vi "HowdyDrive.vi"(6 "highGear?":bool, 8 "error in (no error)":errorcluster, 9 "Y":dbl, 10 "X":dbl, 11 "Drive in":refnum<class "Drive.lvclass">) -> (0 "error out":errorcluster, 3 "Drive out":refnum<class "Drive.lvclass">)   [LabVIEW 2018, in "Drive.lvlib" / "Drive.lvclass"]
doc: "Runs motors based of joystick values in velocity closed loop mode, a version of arcade drive with support for CTRE motor controllers"
uses:
  Drive.lvclass
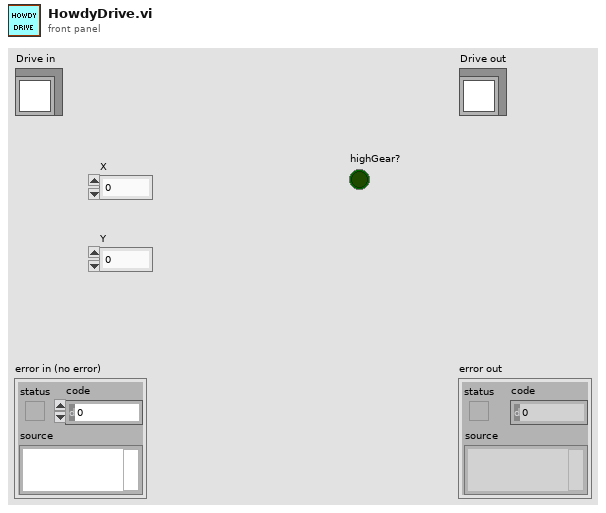
[diagram p1: front panel]
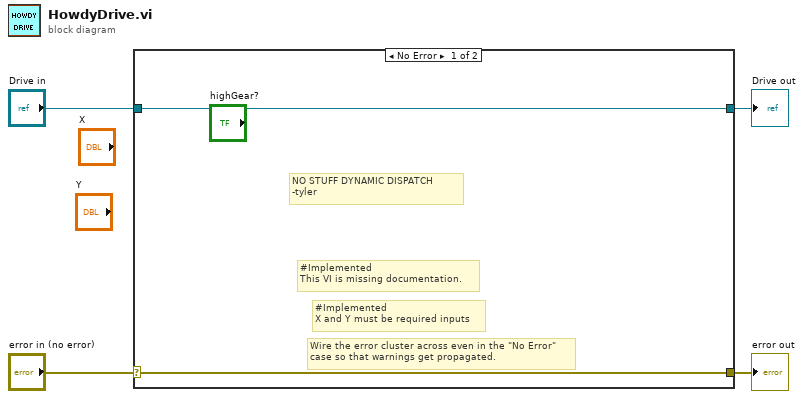
[diagram p0: block diagram]
diagram:
  n1 = case shown="No Error" "error in (no error)" {
    selector: "error in (no error)" -> [w5 w8]
    tunnel: [w5 w8] -> w3
    tunnel: [w6 w7] -> w1
    tunnel: "Drive in" -> [w6 w7]
    frame No Error {
      # "#Implemented\nX and Y must be required inputs"
      # "#Implemented\nThis VI is missing documentation."
      # "NO STUFF DYNAMIC DISPATCH\n-tyler"
      # "Wire the error cluster across even in the \"No Error\"\ncase so that warnings get propagated."
    }
    frame Error {
    }
  }
  "error out" <- w3
  "Drive out" <- w1
